vi "Exit.vi"(8 "error in (no error)":errorcluster, 11 "Old State":refnum<class "Numeric.lvclass">) -> (0 "error out":errorcluster, 3 "New State":refnum<class "Numeric.lvclass">)   [LabVIEW 2020, in "Keypad.lvlib" / "Numeric.lvclass"]
doc: "This is an abstract method. Override this method to define the behavior when you leave the state."
uses:
  Numeric.lvclass
  Keypad/Keypad.lvclass
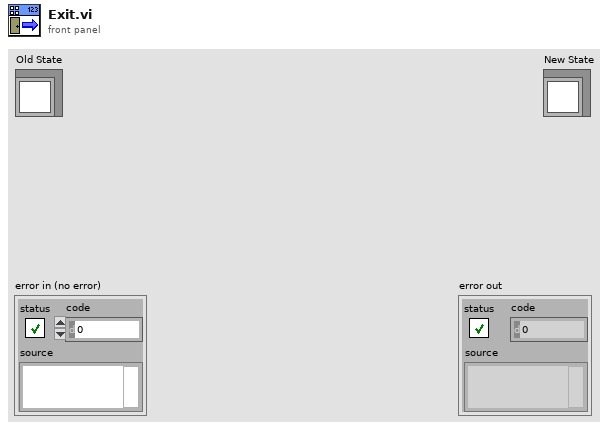
[diagram p1: front panel]
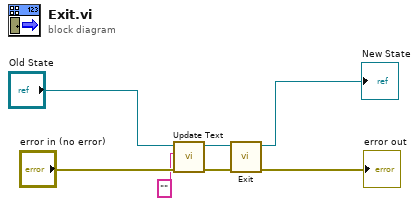
[diagram p0: block diagram]
diagram:
  n1 = call "Update Text.vi"("error in (no error)"="error in (no error)", "Text"="", "Keypad in"="Old State") -> ("error out"=w3:errorcluster, "Keypad out"=w4:refnum<class "Numeric.lvclass">)  [unwired: 7 in]
  n2 = call-parent "Exit.vi"("error in (no error)"=w3, "Old State"=w4) -> ("error out"=→"error out":errorcluster, "New State"=→"New State":refnum<class "Numeric.lvclass">)  [unwired: 8 in]
